vi "Thread@Run__Parameter.vi"(1 "ParamterIn":string) -> (0 "ParamterOut":string)   [LabVIEW 2020]
panel:
  in  "Logic":string(combo)
  in  "Thread":string(combo)="1"
  in  "Index":string(combo)="0"
  in  "Program":string(combo)="1"
  in  "Confirm":bool
  # "Thread@Run $Program(,$ThreadNo ,$Index, $Logic)"
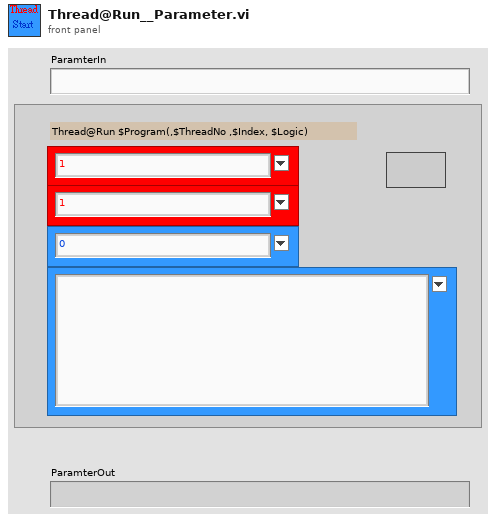
[diagram p1: front panel]
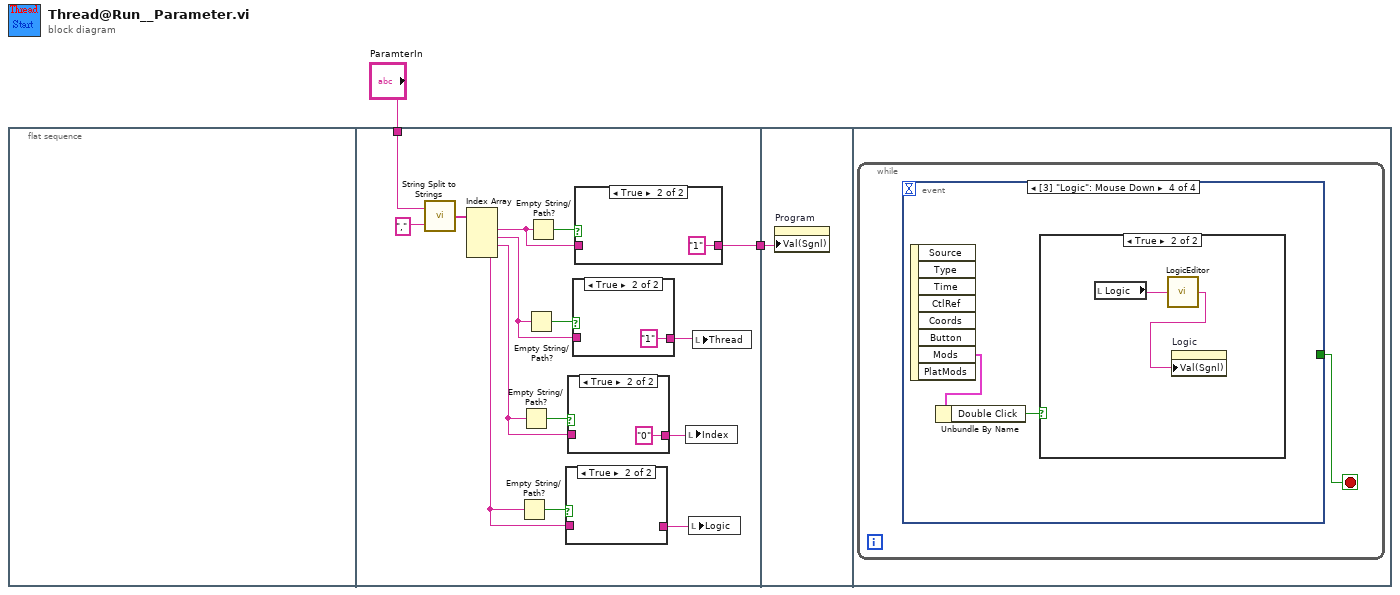
[diagram p0: block diagram]
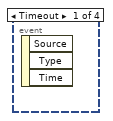
[diagram p6: hidden frame]
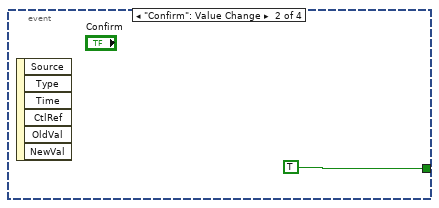
[diagram p7: hidden frame]
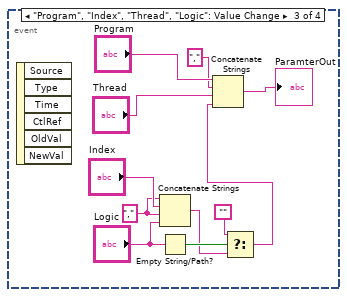
[diagram p8: hidden frame]
diagram:
  n1 = flat-sequence {
    tunnel: "ParamterIn" -> [w15]
    tunnel: [w10] -> w1
    tunnel: w1 -> [w25]
    frame #0 {
    }
    frame #1 {
      n2 = call "String Split to Strings.vi"("search string/char (-)"=",", "String"=w15) -> ("Array"=w17:string[])
      n3 = Index Array(array=w17) -> (element #1=w13:string, element #2=w11:string, element #3=w8:string, element #4=w6:string)  [unwired: 4 in]
      n4 = Empty String/Path?(string/path=w6) -> (empty?=w7:bool)
      n5 = Empty String/Path?(string/path=w8) -> (empty?=w9:bool)
      n6 = Empty String/Path?(string/path=w11) -> (empty?=w12:bool)
      n7 = Empty String/Path?(string/path=w13) -> (empty?=w14:bool)
      n8 = case shown="True" w7 {
        tunnel: w6 -> [w18 _]
        tunnel: [w18 _] -> w5
        frame False {
        }
        frame True {
        }
      }
      n9 = case shown="True" w9 {
        tunnel: w8 -> [w19 _]
        tunnel: [w19 "0"] -> w3
        frame False {
        }
        frame True {
        }
      }
      n10 = case shown="True" w12 {
        tunnel: w11 -> [w21 _]
        tunnel: [w21 "1"] -> w4
        frame False {
        }
        frame True {
        }
      }
      n11 = case shown="True" w14 {
        tunnel: w13 -> [w23 _]
        tunnel: [w23 "1"] -> w10
        frame False {
        }
        frame True {
        }
      }
      n12 = local write "Index"(w3) -> ()
      n13 = local write "Logic"(w5) -> ()
      n14 = local write "Thread"(w4) -> ()
    }
    frame #2 {
      n15 = property on="Program" class="CmbBox"("Val(Sgnl)"=w25) -> ()  [unwired: 2 in, 2 out]
    }
    frame #3 {
      n16 = while {
        stop <- w26 stop-if-true
        n17 = event shown="[3] \"Logic\": Mouse Down" {
          selector: _ -> [_ _ _ _]
          dyn-events: _ -> [_ _ _ _]
          timeout: _ -> [_ _ _ _]
          tunnel: [_ TRUE _ _] -> w26
          event Timeout {
            n18 = event-data() -> ()  [unwired: 1 in, 3 out]
          }
          event "Confirm": Value Change {
            n19 = event-data() -> ()  [unwired: 1 in, 6 out]
          }
          event "Program", "Index", "Thread", "Logic": Value Change {
            w28 = "," ("string")
            n20 = event-data() -> ()  [unwired: 1 in, 6 out]
            n21 = Concatenate Strings(w28, "Index", w28, "Logic") -> (w32:string)
            n22 = Empty String/Path?(string/path="Logic") -> (empty?=w35:bool)
            n23 = Select(t="", s=w35, f=w32) -> (s? t:f=w31:string)
            n24 = Concatenate Strings("Program", "," ("string"), "Thread", w31) -> (→"ParamterOut":string)
          }
          event "Logic": Mouse Down {
            n25 = event-data() -> ("Mods"=w40:cluster{"Double Click":bool, "Menu Key":bool})  [unwired: 1 in, 7 out]
            n26 = Unbundle By Name(w40) -> ("Double Click"=w39:bool)
            n27 = case shown="True" w39 {
              frame False {
              }
              frame True {
                n28 = local read "Logic"() -> (w42:string)
                n29 = call "LogicEditor.vi"("Logic Express"=w42) -> ("LogicExpressOut"=w41:string)
                n30 = property on="Logic" class="CmbBox"("Val(Sgnl)"=w41) -> ()  [unwired: 2 in, 2 out]
              }
            }
          }
        }
      }
    }
  }
